vi "Migrate Global Config.vi"() -> ()   [LabVIEW 2023]
panel:
  out "error out":errorcluster
  in  "error in (no error)":errorcluster
  in  "App Data Directory":path
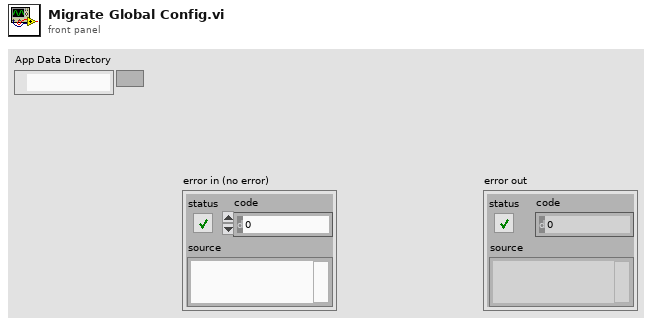
[diagram p1: front panel]
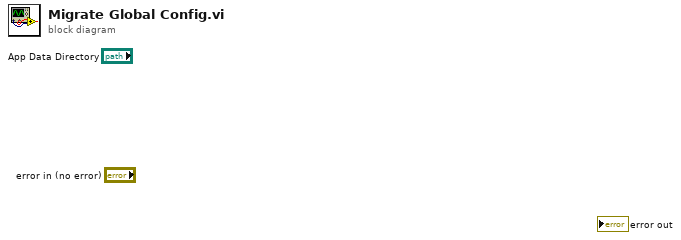
[diagram p0: block diagram]
diagram:
